vi "Read Payload.vi"(11 "ActionStack in":refnum<class "Stack.lvclass">) -> (2 "Payload":variant, 3 "ActionStack out":refnum<class "Stack.lvclass">)   [LabVIEW 2025]
uses:
  Stack.lvclass/Stack.ctl
  Stack.lvclass
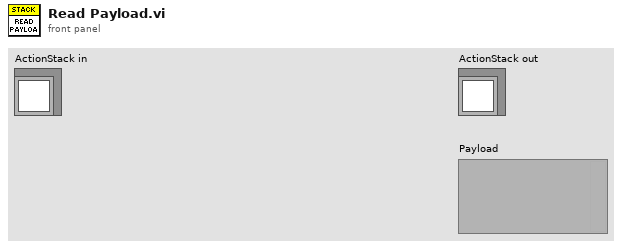
[diagram p1: front panel]
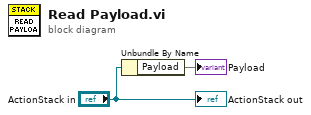
[diagram p0: block diagram]
diagram:
  n1 = Unbundle By Name("ActionStack in") -> ("Payload"=→"Payload")
  "ActionStack out" <- "ActionStack in"
